vi "Abort Multipart Upload.vi"(4 "Region":T1, 8 "error in (no error)":errorcluster, 11 "Multipart Upload RefNum in":T2) -> (0 "error out":errorcluster, 2 "No Such Upload":bool, 3 "Multipart Upload RefNum out":T2)   [LabVIEW 2015, in "LV Interface for Amazon S3.lvlib"]
doc: "This operation <B>aborts a multipart upload</B>. After a multipart upload is aborted, <B>no additional parts can be uploaded using that multipart upload reference</B>. The <B>storage consumed</B> by any previously uploaded parts <B>will be freed</B>. However, <B>if any part uploads are currently in progress, those</B> part uploads <B>might or might not succeed</B>. As a result, <B>it might be necessary to abort a given multipart upload multiple times</B> in order to completely free all storage consumed by all parts."
uses:
  LV Interface for Amazon S3.lvlib
  Typedefs/AMZ_S3_Multipart Upload RefNum.ctl
  Typedefs/AMZ_S3_Multipart Upload RefNum Enum.ctl
  Typedefs/AMZ_S3_LocationConstraint.ctl
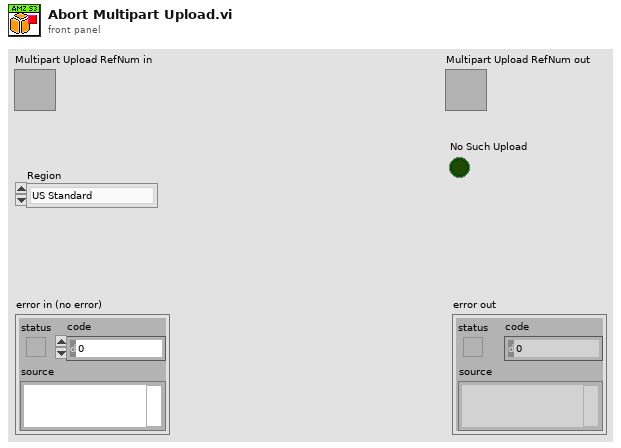
[diagram p1: front panel]
types:
  T1 = typedef "LV Interface for Amazon S3.lvlib/AMZ_S3_LocationConstraint.ctl" = enum16{"US Standard", "us-east-2", "us-west-1", "us-west-2", "ap-northeast-1", "ap-northeast-2", "ap-southeast-1", "ap-southeast-2", "ca-central-1", "eu-central-1", "eu-west-1", "eu-west-2", "sa-east-1"}
  T2 = typedef "LV Interface for Amazon S3.lvlib/AMZ_S3_Multipart Upload RefNum.ctl" = refnum<k1>
  T3 = typedef "LV Interface for Amazon S3.lvlib/AMZ_S3_Multipart Upload Data.ctl" = cluster{"Object":string, "Bucket":string, "UploadID":string, "Parts":T4[]}
  T4 = typedef "LV Interface for Amazon S3.lvlib/AMZ_S3_Multipart Upload Part Data.ctl" = cluster{"PartNumber":u16, "Lat modified":timestamp, "ETag":string, "Size":u64}
  T5 = cluster{"format string":string, "UploadID":string}
  T6 = cluster{"format string":string, "UploadID":string}[]
  T7 = typedef "LV Interface for Amazon S3.lvlib/AMZ_S3_Call Results.ctl" = enum16{"Success", "UndefinedError", "AccessDenied", "AccountProblem", "AmbiguousGrantByEmailAddress", "BadDigest", "BucketAlreadyExists", "BucketAlreadyOwnedByYou", "BucketNotEmpty", "CredentialsNotSupported", "CrossLocationLoggingProhibited", "EntityTooSmall", "EntityTooLarge", "ExpiredToken", "IllegalVersioningConfigurationException", "IncompleteBody", "IncorrectNumberOfFilesInPostRequest", "InlineDataTooLarge", "InternalError", "InvalidAccessKeyId", "InvalidAddressingHeader", "InvalidArgument", "InvalidBucketName", "InvalidDigest", "InvalidLocationConstraint", "InvalidPart", "InvalidPartOrder", "InvalidPayer", "InvalidPolicyDocument", "InvalidRange", "InvalidSecurity", "InvalidSOAPRequest", "InvalidStorageClass", "InvalidTargetBucketForLogging", "InvalidToken", "InvalidURI", "KeyTooLong", "MalformedACLError", "MalformedPOSTRequest", "MalformedXML", "MaxMessageLengthExceeded", "MaxPostPreDataLengthExceededError", "MetadataTooLarge", "MethodNotAllowed", "MissingAttachment", "MissingContentLength", "MissingRequestBodyError", "MissingSecurityElement", "MissingSecurityHeader", "NoLoggingStatusForKey", "NoSuchBucket", "NoSuchKey", "NoSuchUpload", "NoSuchVersion", "NotImplemented", "NotSignedUp", "OperationAborted", "PermanentRedirect", "PreconditionFailed", "Redirect", "RequestIsNotMultiPartContent", "RequestTimeout", "RequestTimeTooSkewed", "RequestTorrentOfBucketError", "SignatureDoesNotMatch", "SlowDown", "TemporaryRedirect", "TokenRefreshRequired", "TooManyBuckets", "UnexpectedContent", "UnresolvableGrantByEmailAddress", "UserKeyMustBeSpecified", "LabVIEWError"}
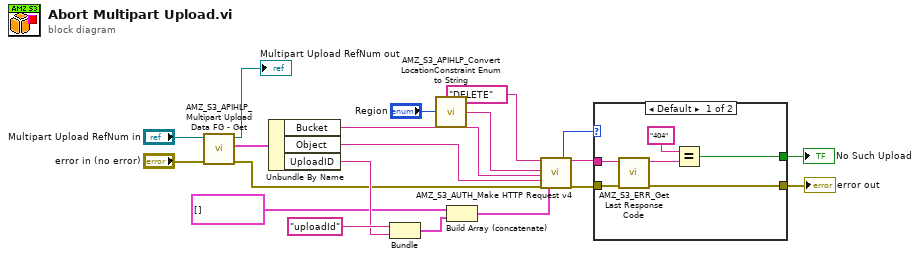
[diagram p0: block diagram]
diagram:
  n1 = call "AMZ_S3_APIHLP_Multipart Upload Data FG - Get.vi"("error in (no error)"="error in (no error)", "Multipart Upload RefNum in"="Multipart Upload RefNum in") -> ("error out"=w7:errorcluster, "Multipart Upload Data"=w18:T3, "Multipart Upload RefNum out"=→"Multipart Upload RefNum out":T2)  [unwired: 7 in]
  n2 = Unbundle By Name(w18) -> ("Bucket"=w4:string, "Object"=w5:string, "UploadID"=w13:string)
  n3 = Bundle("format string"="uploadId", "UploadID"=w13) -> (w12:T5)  [unwired: 1 in]
  n4 = call "AMZ_S3_APIHLP_Convert LocationConstraint Enum to String.vi"("Location"="Region") -> ("Location String"=w2:string)  [unwired: 4 in]
  n5 = Build Array (concatenate)(cluster{"item":string, "value":string}[] [] ("request parameters"), w12) -> (w6:T6)
  n6 = call "AMZ_S3_AUTH_Make HTTP Request v4.vi"("HTTP-Verb"="DELETE", "Region"=w2, "Bucket"=w4, "Object Key"=w5, "error in"=w7, "request parameters"=w6) -> ("Call Result"=w9:T7, "response headers"=w10:string, "error out"=w8:errorcluster)  [unwired: 10 in, 1 out]
  n7 = case shown="Default" w9 {
    tunnel: w8 -> [w26 w27]
    tunnel: w10 -> [w25 _]
    tunnel: [w21 w27] -> w16
    tunnel: [w22 _] -> w15
    frame Default {
      n8 = call "AMZ_S3_ERR_Get Last Response Code.vi"("error in (no error)"=w26, "Response header"=w25) -> ("error out"=w21:errorcluster, "Response code (last)"=w24:string)  [unwired: 8 in]
      n9 = Equal?(x="404", y=w24) -> (x = y?=w22:bool)
    }
    frame "Success" {
    }
  }
  "error out" <- w16
  "No Such Upload" <- w15
